vi "New Data Logging Specification (TDMS).vi"(5 "File Properties":T3[](array[typedef]), 6 "Apply Root Properties to Groups":bool, 7 "File Description":string, 8 "error in (no error)":errorcluster, 9 "Channel Groups":T2[](array[typedef]), 10 "File Conflict Operation":T1, 11 "Base Log File Path":path) -> (0 "error out":errorcluster, 3 "Data Logging Specification Ref out":T6)   [LabVIEW 2020, in "NI_VS Data Logging API.lvlib"]
doc: "Creates a new data logging specification, which defines the channels to log and the type and base path for log files. You can log data to TDMS or text (.txt) files. You must manually select the polymorphic instance to use."
uses:
  <vilib>/NI VeriStand/Execution/DataLogging/NI_VS Data Logging API.lvlib
  <vilib>/NI VeriStand/Execution/DataLogging/DataLoggingSpecification Ref.ctl
  NationalInstruments.VeriStand.ClientAPI
  <vilib>/NI VeriStand/Execution/DataLogging/TDMS Property.ctl
  <vilib>/NI VeriStand/Execution/DataLogging/TDMS Channel Group.ctl
  <vilib>/NI VeriStand/Execution/DataLogging/TDMS Channel.ctl
  <vilib>/NI VeriStand/Execution/DataLogging/Time Channel Options.ctl
  <vilib>/NI VeriStand/Execution/DataLogging/File Conflict Operation.ctl
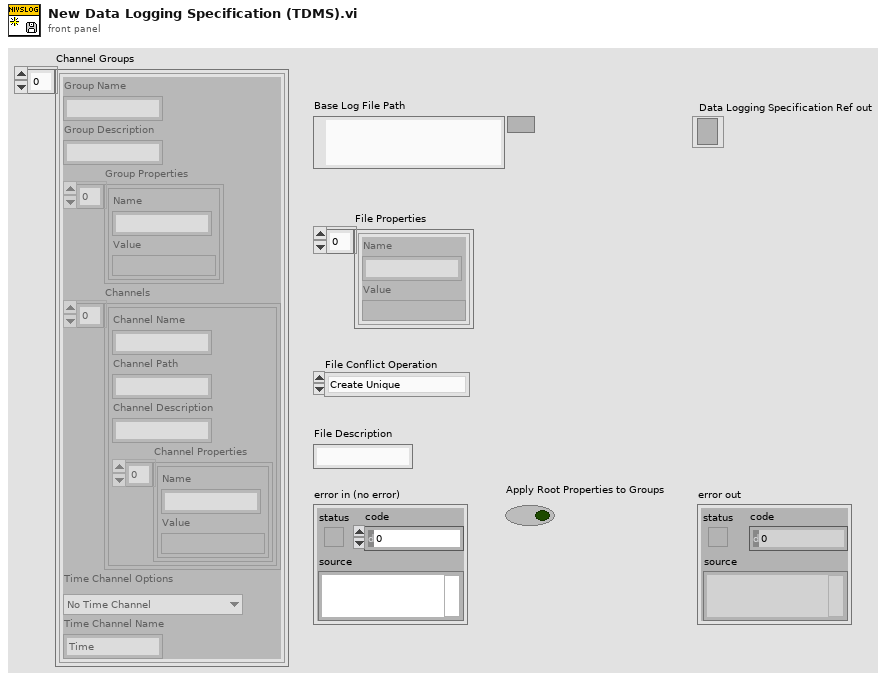
[diagram p1: front panel]
types:
  T1 = typedef "NI_VS Data Logging API.lvlib/File Conflict Operation.ctl" = enum16{"Create Unique", "Append to Existing", "Overwrite"}
  T2 = typedef "NI_VS Data Logging API.lvlib/TDMS Channel Group.ctl" = cluster{"Group Name":string, "Group Description":string, "Group Properties":T3[], "Channels":T4[], "Time Channel Options":T5, "Time Channel Name":string}
  T3 = typedef "NI_VS Data Logging API.lvlib/TDMS Property.ctl" = cluster{"Name":string, "Value":variant}
  T4 = typedef "NI_VS Data Logging API.lvlib/TDMS Channel.ctl" = cluster{"Channel Name":string, "Channel Path":string, "Channel Description":string, "Channel Properties":T3[]}
  T5 = typedef "NI_VS Data Logging API.lvlib/Time Channel Options.ctl" = enum16{"No Time Channel", "Absolute Time", "System Time", "System Time - Microseconds", "Absolute Time as Double", "Relative To First Start Trigger", "Relative To Session Start"}
  T6 = typedef "NI_VS Data Logging API.lvlib/DataLoggingSpecification Ref.ctl" = refnum<k24>
  T7 = typedef "NI_VS Data Logging API.lvlib/TdmsLogFile Ref.ctl" = refnum<k24>
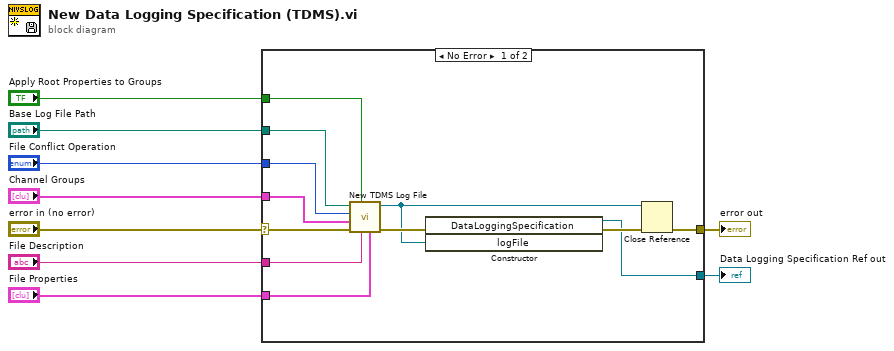
[diagram p0: block diagram]
diagram:
  n1 = case shown="No Error" "error in (no error)" {
    selector: "error in (no error)" -> [w16 w22]
    tunnel: [w18 _] -> w8
    tunnel: [w17 w22] -> w7
    tunnel: "File Description" -> [w15 _]
    tunnel: "File Properties" -> [w14 _]
    tunnel: "Channel Groups" -> [w13 _]
    tunnel: "File Conflict Operation" -> [w12 _]
    tunnel: "Base Log File Path" -> [w11 _]
    tunnel: "Apply Root Properties to Groups" -> [w10 _]
    frame No Error {
      n2 = call <vilib>:"New TDMS Log File.vi"("File Properties"=w14, "File Description"=w15, "Apply Root Properties to Groups"=w10, "error in (no error)"=w16, "Channel Groups"=w13, "File Conflict Operation"=w12, "Log File Path"=w11) -> ("error out"=w21:errorcluster, "TDMSLogFile Ref"=w19:T7)  [unwired: 3 in]
      n3 = constructor class="DataLoggingSpecification"(error in=w21, "logFile"=w19) -> (reference out=w18:refnum<k24>, error out=w20:errorcluster)  [unwired: 2 in, 2 out]
      n4 = Close Reference(reference=w19, error in (no error)=w20) -> (error out=w17:errorcluster)
    }
    frame Error {
    }
  }
  "error out" <- w7
  "Data Logging Specification Ref out" <- w8
